vi "GetParam.vi"(8 "error in (no error)":errorcluster caption="entrée d'erreur (pas d'erreur)", 11 "FeatureHasher.lvclass":refnum<class "FeatureHasher.lvclass">) -> (0 "error out":errorcluster caption="sortie d'erreur", 2 "FeatureHasher":T1={"n_features"=1048576, "input_type"="dict", "dtype"="float", "alternate_sign"=TRUE}, 3 "FeatureHasher.lvclass":refnum<class "FeatureHasher.lvclass">)   [LabVIEW 2020, in "FeatureHasher.lvclass"]
doc: "Get Parameters"
uses:
  FeatureHasher.lvclass
  FeatureHasher.lvclass/FeatureHasher.ctl
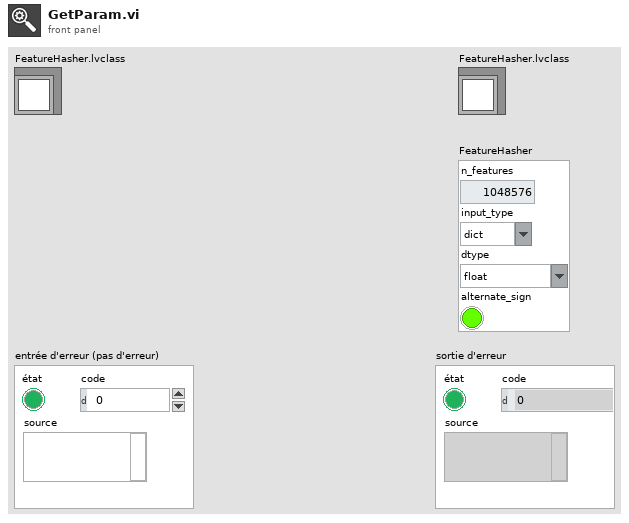
[diagram p1: front panel]
types:
  T1 = cluster{"n_features":i32, "input_type":string, "dtype":string, "alternate_sign":bool}
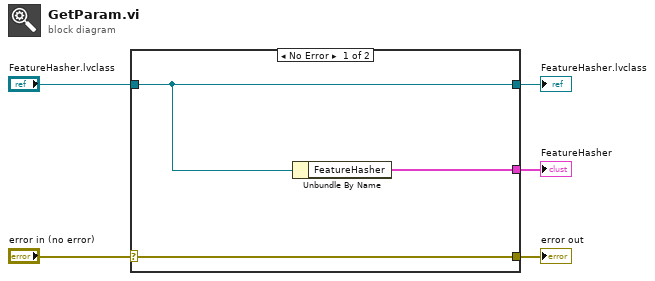
[diagram p0: block diagram]
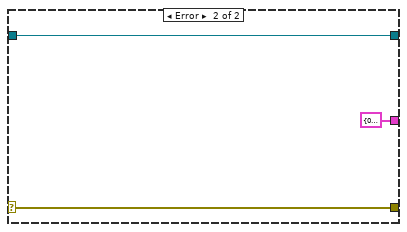
[diagram p2: hidden frame]
diagram:
  n1 = case shown="No Error" "error in (no error)" {
    selector: "error in (no error)" -> [w8 w10]
    tunnel: [w8 w10] -> w4
    tunnel: [w7 w11] -> w2
    tunnel: "FeatureHasher.lvclass" -> [w7 w11]
    tunnel: [w6 T1 {"n_features"=0, "input_type"="", "dtype"="", "alternate_sign"=FALSE} ("FeatureHasher")] -> w1
    frame No Error {
      n2 = Unbundle By Name(w7) -> ("FeatureHasher"=w6:T1)
    }
    frame Error {
    }
  }
  "error out" <- w4
  "FeatureHasher.lvclass" <- w2
  "FeatureHasher" <- w1
